vi "IsErrorCluster.vi"(9 "Cluster Elements":variant[](array[variant])) -> (3 "Boolean":bool)   [LabVIEW 2020]
uses:
  <vilib>/Utility/VariantDataType/VariantType.lvlib
panel:
  out "error IO":errorcluster
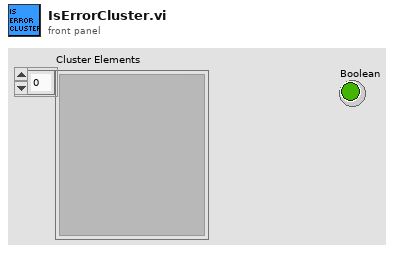
[diagram p1: front panel]
types:
  T1 = typedef "LVNumericRepresentation.ctl" = enum32{"Extended Precision", "Double Precision", "Single Precision", "Long", "Word", "Byte", "Unsigned Long", "Unsigned Word", "Unsigned Byte", "Complex Extended", "Complex Double", "Complex Single", "Quad", "Unsigned Quad", "Fixed-Point"}
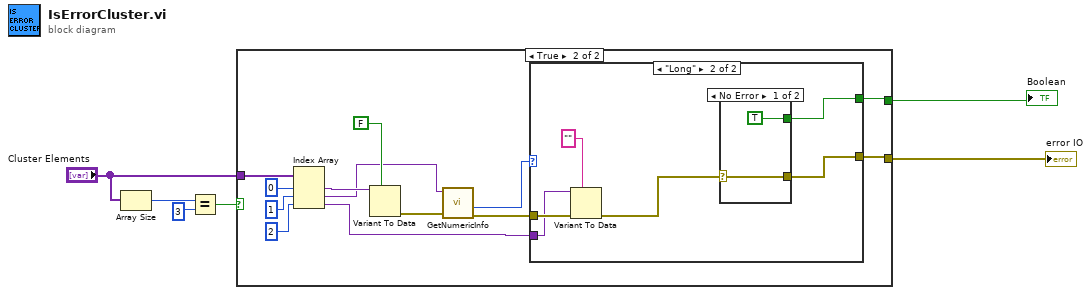
[diagram p0: block diagram]
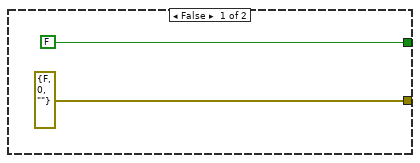
[diagram p2: hidden frame]
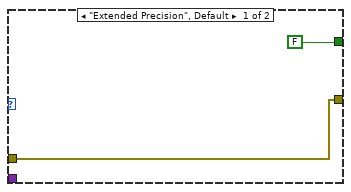
[diagram p3: hidden frame]
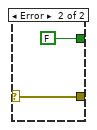
[diagram p4: hidden frame]
diagram:
  n1 = Array Size(array="Cluster Elements") -> (size(s)=w5:i32)
  n2 = Equal?(x=w5, y=3) -> (x = y?=w6:bool)
  n3 = case shown="True" w6 {
    tunnel: "Cluster Elements" -> [_ w21]
    tunnel: [errorcluster {"status"=FALSE, "code"=0, "source"=""} ("error IO") w17] -> w2
    tunnel: [FALSE w16] -> w1
    frame False {
    }
    frame True {
      n4 = Index Array(array=w21, index #1=0 ("index"), index #2=1 ("index"), index #3=2 ("index")) -> (element #1=w15:variant, element #2=w12:variant, element #3=w9:variant)
      n5 = Variant To Data(type=FALSE ("status"), Variant=w15) -> (error out=w13:errorcluster)  [unwired: 1 in, 1 out]
      n6 = call <vilib>:"GetNumericInfo.vi"("error in (no error)"=w13, "Variant"=w12) -> ("error out"=w11:errorcluster, "representation"=w10:T1)  [unwired: 6 in, 2 out]
      n7 = case shown="\"Long\"" w10 {
        tunnel: [w22 w29] -> w17
        tunnel: [FALSE w28] -> w16
        tunnel: w11 -> [w22 w27]
        tunnel: w9 -> [_ w25]
        frame "Extended Precision", Default {
        }
        frame "Long" {
          n8 = Variant To Data(error in=w27, type="" ("source"), Variant=w25) -> (error out=w26:errorcluster)  [unwired: 1 out]
          n9 = case shown="No Error" w26 {
            selector: w26 -> [w31 w33]
            tunnel: [w31 w33] -> w29
            tunnel: [TRUE FALSE] -> w28
            frame No Error {
            }
            frame Error {
            }
          }
        }
      }
    }
  }
  "error IO" <- w2
  "Boolean" <- w1
